vi "Untitled 1.vi"() -> ()   [LabVIEW 2012]
panel:
  out "Waveform Graph 2":dbl[][](graph)
  in  "y":i32
  in  "stop":bool
  in  "Total Delta C1(pF)":string[](array[string])=["6.607E+0", "6.594E+0", "6.484E+0", "6.152E+0", "6.274E+0", "6.287E+0", "6.049E+0", "6.185E+0", "2.000E-6", "-201.000E-6", "-2.382E-3", "-178.000E-6", "2.508E-3", "-75.000E-6", "58.000E-6", "1.293E-3"]
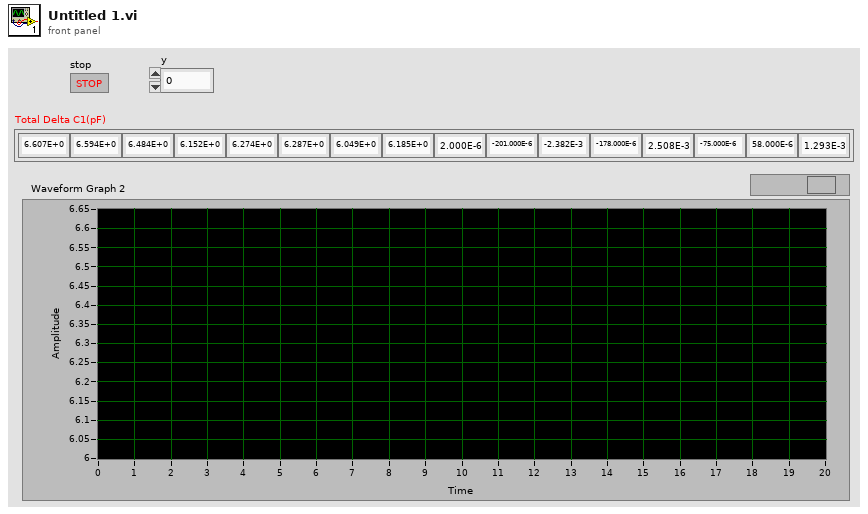
[diagram p1: front panel]
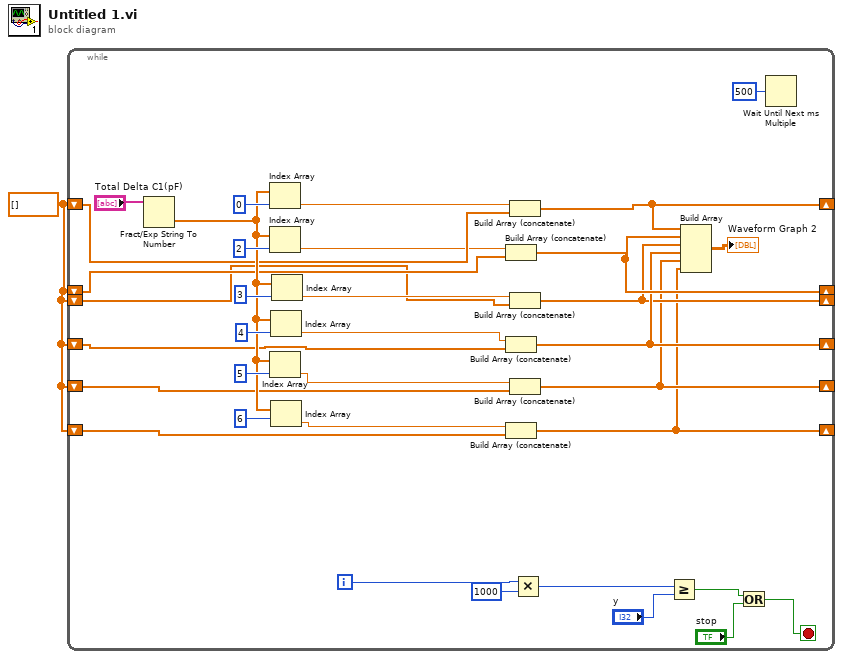
[diagram p0: block diagram]
diagram:
  w1 = dbl[] []
  n1 = while {
    shift-right: [w20] -> _
    shift-left: w1 -> [w23]
    shift-right: [w18] -> _
    shift-left: w1 -> [w13]
    shift-right: [w12] -> _
    shift-left: w1 -> [w11]
    shift-right: [w10] -> _
    shift-left: w1 -> [w9]
    shift-right: [w7] -> _
    shift-left: w1 -> [w8]
    shift-right: [w5] -> _
    shift-left: w1 -> [w6]
    i -> [w4]
    stop <- w26 stop-if-true
    n2 = Fract/Exp String To Number(string="Total Delta C1(pF)") -> (number=w24:dbl[])  [unwired: 3 in, 1 out]
    n3 = Index Array(array=w24, index=0) -> (element=w22:dbl)
    n4 = Index Array(array=w24, index=2) -> (element=w21:dbl)
    n5 = Index Array(array=w24, index=5) -> (element=w15:dbl)
    n6 = Index Array(array=w24, index=4) -> (element=w16:dbl)
    n7 = Index Array(array=w24, index=6) -> (element=w14:dbl)
    n8 = Index Array(array=w24, index=3) -> (element=w17:dbl)
    n9 = Build Array (concatenate)(w21, w13) -> (w18:dbl[])
    n10 = Build Array (concatenate)(w16, w11) -> (w12:dbl[])
    n11 = Build Array (concatenate)(w14, w6) -> (w5:dbl[])
    n12 = Build Array (concatenate)(w22, w23) -> (w20:dbl[])
    n13 = Build Array (concatenate)(w17, w9) -> (w10:dbl[])
    n14 = Build Array (concatenate)(w15, w8) -> (w7:dbl[])
    n15 = Multiply(x=w4, y=1000) -> (x*y=w2:i32)
    n16 = Greater Or Equal?(x=w2, y="y") -> (x >= y?=w28:bool)
    n17 = Build Array(w20, w18, w10, w12, w7, w5) -> (→"Waveform Graph 2":dbl[][])
    n18 = Or(x=w28, y="stop") -> (x .or. y?=w26:bool)
    n19 = Wait Until Next ms Multiple(millisecond multiple=u32 500) -> ()  [unwired: 1 out]
  }
